vi "tb_Multiply Float.vi"() -> ()   [LabVIEW 2011]
panel:
  out "Array":sgl[](array[numeric])
  out "Output Valid":bool[](array[boolean])
  in  "Input 2":sgl
  in  "Input 1":sgl
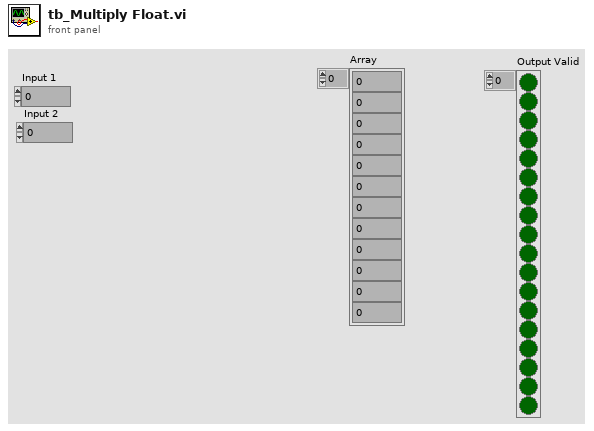
[diagram p1: front panel]
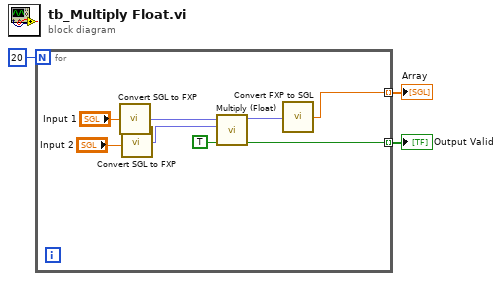
[diagram p0: block diagram]
diagram:
  n1 = for {
    N: 20 -> [_]
    tunnel: [w6] -> w3 mode=indexing
    tunnel: [w4] -> w1 mode=indexing
    n2 = call <userlib>:"Convert SGL to FXP.vi"("Input"="Input 1") -> ("FXP Output"=w11:fxp<+,32,32>)  [unwired: 14 in]
    n3 = call <userlib>:"Convert SGL to FXP.vi"("Input"="Input 2") -> ("FXP Output"=w10:fxp<+,32,32>)  [unwired: 14 in]
    n4 = call <userlib>:"Multiply (Float).vi"("Input Valid"=TRUE, "b"=w10, "a"=w11) -> ("Output Valid"=w6:bool, "a*b"=w5:fxp<+,32,32>)  [unwired: 7 in]
    n5 = call <userlib>:"Convert FXP to SGL.vi"("FXP Input"=w5) -> ("Output SGL"=w4:sgl)  [unwired: 14 in]
  }
  "Output Valid" <- w3
  "Array" <- w1
